vi "COM UUT Board.vi"(8 "error in (no error)":errorcluster, 10 "VI reference (current VI)":refnum<vi>, 11 "VISA resource name 2":refnum<visa-resource-name>) -> (0 "error out":errorcluster, 2 ".not. x?":bool, 3 "VISA resource name out":refnum<visa-resource-name>)   [LabVIEW 2017]
uses:
  <vilib>/Instr/_visa.llb/VISA Configure Serial Port (Instr).vi
panel:
  in  "Blank Button":bool
  in  "VISA resource name":refnum<visa-resource-name>
  # "Please choose the UUT COM Port"
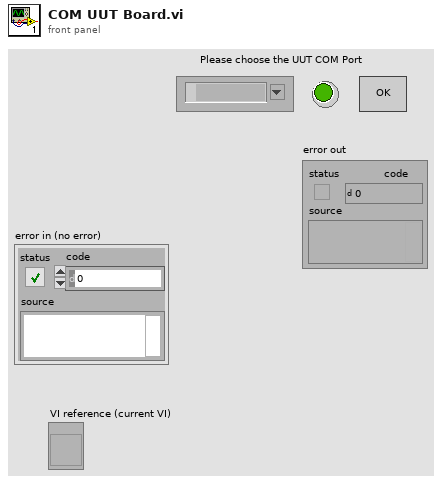
[diagram p1: front panel]
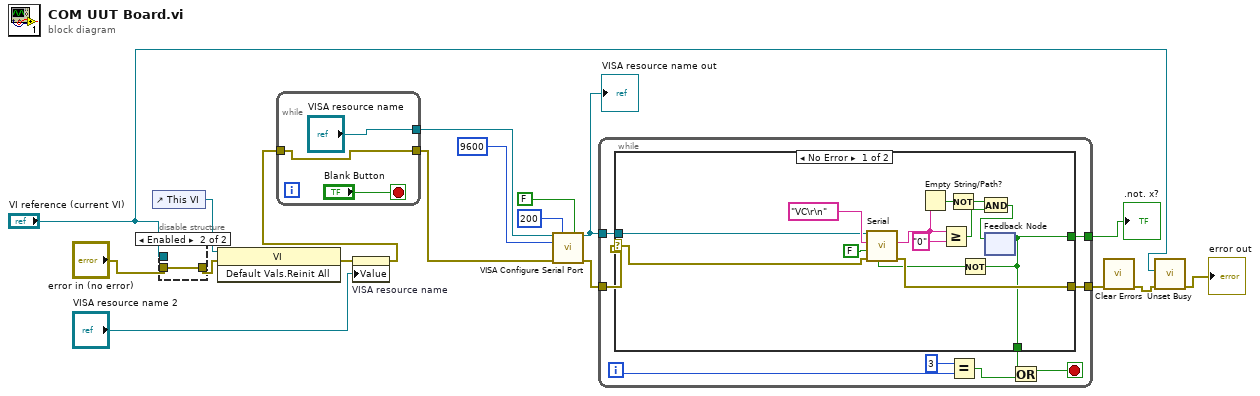
[diagram p0: block diagram]
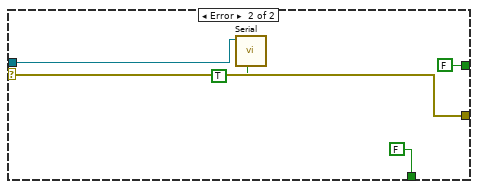
[diagram p2: hidden frame]
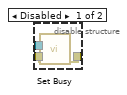
[diagram p3: hidden frame]
diagram:
  n1 = control-ref of="This VI"() -> (w18:refnum<vi>)
  n2 = disable-structure shown="Enabled" {
    disable-tunnel: "VI reference (current VI)" -> [w21 _]
    disable-tunnel: "error in (no error)" -> [w20 w22]
    disable-tunnel: [w19 w22] -> w5
    frame Disabled {
      n3 = call <vilib>:"Set Busy.vi"("error in (no error)"=w20, "VI reference (current VI)"=w21) -> ("error out"=w19:errorcluster)  [unwired: 8 in, 1 out]
    }
    frame Enabled {
    }
  }
  n4 = invoke class="VI" method="Default Vals.Reinit All"(reference=w18, error in=w5) -> (error out=w17:errorcluster)  [unwired: 1 in, 2 out]
  n5 = property on="VISA resource name" class="VISAName"(error in=w17, "Value"="VISA resource name 2") -> (error out=w4:errorcluster)  [unwired: 1 in, 1 out]
  n6 = while {
    tunnel: ["VISA resource name"] -> w15
    tunnel: w4 -> [w23]
    tunnel: [w23] -> w3
    stop <- "Blank Button" stop-if-true
  }
  n7 = call-poly "VISA Configure Serial Port"("VISA resource name"=w15, "timeout (10sec)"=u32 200, "Enable Termination\nChar (T)"=FALSE ("Enable Termination\nChar (T)"), "baud rate (9600)"=u32 9600 ("baud rate"), "error in (no error)"=w3) -> ("VISA resource name out"=w12:refnum<visa-resource-name>, "error out"=w8:errorcluster)  [unwired: 9 in]
  "VISA resource name out" <- w12
  n8 = while {
    tunnel: w12 -> [w34]
    tunnel: [w32] -> w9
    tunnel: w8 -> [w31]
    tunnel: [w33] -> w11
    i -> [w28]
    stop <- w29 stop-if-true
    n9 = case shown="No Error" w31 {
      selector: w31 -> [w42 w51]
      tunnel: w34 -> [w44 w49]
      tunnel: [w43 w51] -> w33
      tunnel: [w41 FALSE] -> w32
      tunnel: [w41 FALSE] -> w30
      frame No Error {
        n10 = feedback #1() -> (w41:bool)  [unwired: 1 in]
        n11 = Not(x=w41) -> (.not. x?=w40:bool)
        n12 = call "Serial.vi"("Close"=w40, "error in (no error)"=w42, "Clear Log"=FALSE, "write buffer"="VC\r\n", "VISA resource name"=w44) -> ("error out"=w43:errorcluster, "read buffer"=w39:string)  [unwired: 5 in]
        n13 = Empty String/Path?(string/path=w39) -> (empty?=w36:bool)
        n14 = Greater Or Equal?(x=w39, y="0") -> (x >= y?=w38:bool)
        n15 = Not(x=w36) -> (.not. x?=w35:bool)
        n16 = And(x=w35, y=w38) -> (x .and. y?=w37:bool)
        n17 = feedback-in #1(w37) -> ()
      }
      frame Error {
        n18 = call "Serial.vi"("Close"=TRUE, "VISA resource name"=w49) -> ()  [unwired: 8 in, 2 out]
      }
    }
    n19 = Equal?(x=3, y=w28) -> (x = y?=w26:bool)
    n20 = Or(x=w30, y=w26) -> (x .or. y?=w29:bool)
  }
  ".not. x?" <- w9
  n21 = call <vilib>:"Clear Errors.vi"("error in (no error)"=w11) -> ("error out"=w10:errorcluster)  [unwired: 5 in, 1 out]
  n22 = call <vilib>:"Unset Busy.vi"("error in (no error)"=w10, "VI reference (current VI)"="VI reference (current VI)") -> ("error out"=→"error out":errorcluster)  [unwired: 9 in]
